vi "TCam_CenterArray.vi"(4 "draw all?":bool, 5 "Size":u32, 6 "Point Array":T2[](array[typedef]) {"Y" format="%.2f"; "X" format="%.2f"}, 7 "Image in":T1) -> (0 "Array":cluster{"X":i32, "Y":i32}[][](array[cluster]), 1 "Image":T1(plugin-control))   [LabVIEW 2022 SP3]
uses:
  <vilib>/vision/Image Controls.llb/IMAQ Image.ctl
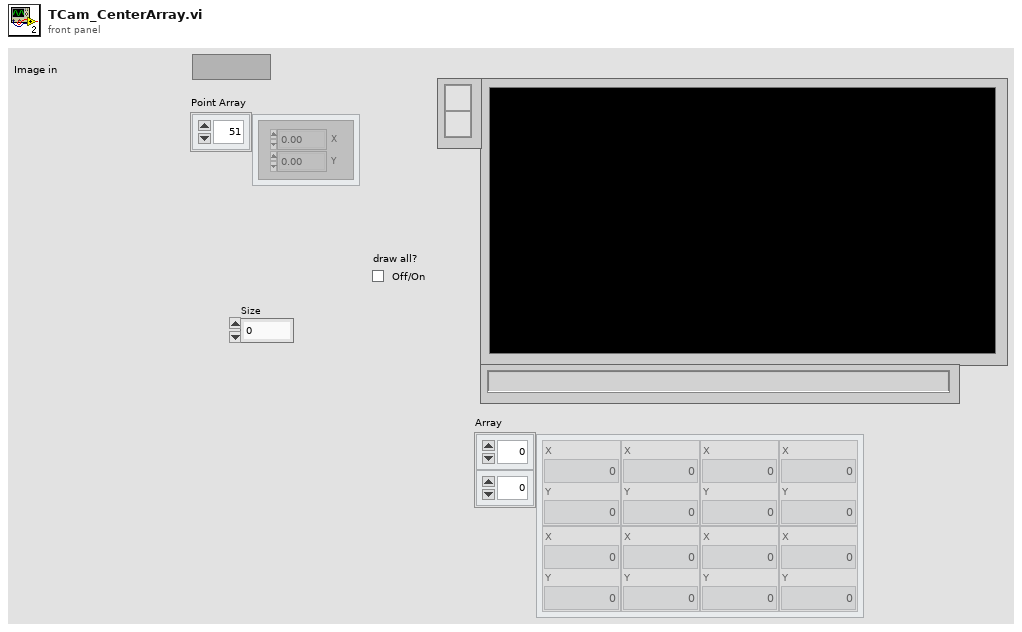
[diagram p1: front panel]
types:
  T1 = typedef "IMAQ Image.ctl" = refnum<image>
  T2 = typedef "IMAQ Point" = cluster{"X":sgl, "Y":sgl}
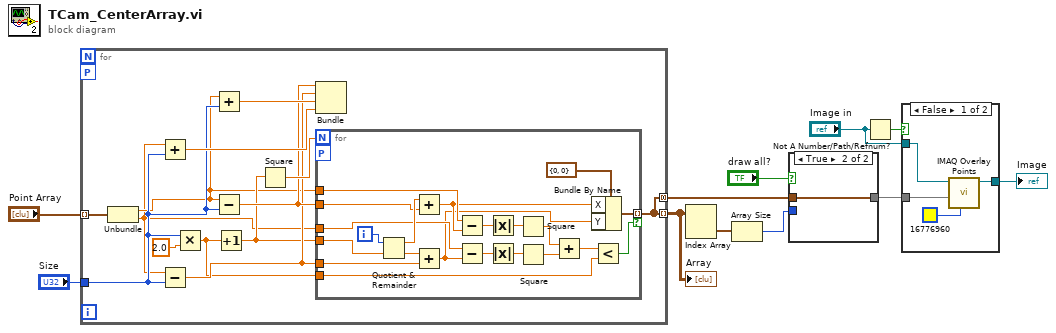
[diagram p0: block diagram]
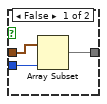
[diagram p3: hidden frame]
diagram:
  n1 = for {
    tunnel: "Size" -> [w22]
    tunnel: "Point Array" -> [w17] mode=indexing
    tunnel: [w12] -> w5 mode=indexing
    tunnel: [w12] -> w7 mode=concatenating
    workers-P: _ -> [_]
    n2 = Unbundle(w17) -> ("X"=w15:sgl, "Y"=w14:sgl)
    n3 = Add(x=w14, y=w22) -> (x+y=w23:sgl)
    n4 = Subtract(x=w14, y=w22) -> (x-y=w18:sgl)
    n5 = Multiply(x=w22, y=2.0) -> (x*y=w13:dbl)
    n6 = Add(x=w15, y=w22) -> (x+y=w24:sgl)
    n7 = Subtract(x=w15, y=w22) -> (x-y=w19:sgl)
    n8 = Increment(x=w13) -> (x+1=w16:dbl)
    n9 = Square(x=w16) -> (x^2=w20:dbl)
    n10 = Bundle(w19, w18, w24, w23) -> ()  [unwired: 1 in, 1 out]
    n11 = for {
      N: w20 -> [_]
      tunnel: w16 -> [w44]
      tunnel: w19 -> [w42]
      tunnel: w18 -> [w40]
      tunnel: [w39] -> w12 mode=indexing if=w25
      tunnel: w15 -> [w37]
      tunnel: w14 -> [w30]
      tunnel: w13 -> [w26]
      workers-P: _ -> [_]
      i -> [w45]
      n12 = Quotient & Remainder(x=w45, y=w44) -> (x-y*floor(x/y)=w43:dbl, floor(x/y)=w41:dbl)
      n13 = Add(x=w43, y=w42) -> (x+y=w36:dbl)
      n14 = Add(x=w41, y=w40) -> (x+y=w29:dbl)
      n15 = Subtract(x=w37, y=w36) -> (x-y=w35:dbl)
      n16 = Subtract(x=w30, y=w29) -> (x-y=w32:dbl)
      n17 = Absolute Value(x=w35) -> (abs(x)=w34:dbl)
      n18 = Absolute Value(x=w32) -> (abs(x)=w31:dbl)
      n19 = Square(x=w34) -> (x^2=w33:dbl)
      n20 = Square(x=w31) -> (x^2=w28:dbl)
      n21 = Add(x=w33, y=w28) -> (x+y=w27:dbl)
      n22 = Bundle By Name(cluster=cluster{"X":i32, "Y":i32} {"X"=0, "Y"=0} ("Point"), "X"=w36, "Y"=w29) -> (w39:cluster{"X":i32, "Y":i32})
      n23 = Less?(x=w27, y=w26) -> (x < y?=w25:bool)
    }
  }
  "Array" <- w5
  n24 = Index Array(array=w5) -> (element=w4:cluster{"X":i32, "Y":i32}[])  [unwired: 2 in]
  n25 = Array Size(array=w4) -> (size(s)=w3:i32)
  n26 = case shown="True" "draw all?" {
    tunnel: [w46 w49] -> w8
    tunnel: w7 -> [w48 w49]
    tunnel: w3 -> [w47 _]
    frame False {
      n27 = Array Subset(array=w48, length=w47) -> (w46:cluster{"X":i32, "Y":i32}[])  [unwired: 1 in]
    }
    frame True {
    }
  }
  n28 = Not A Number/Path/Refnum?(number/path/refnum="Image in") -> (NaN/Path/Refnum?=w1:bool)
  n29 = case shown="False" w1 {
    tunnel: [w53 w54] -> w9
    tunnel: w8 -> [w51 _]
    tunnel: "Image in" -> [w50 w54]
    frame False {
      n30 = call "IMAQ Overlay Points"("Color"=u32 16776960, "Array of Points"=w51, "Image"=w50) -> ("Image Out"=w53:T1)  [unwired: 7 in, 1 out]
    }
    frame True {
    }
  }
  "Image" <- w9
